vi "AO FIFO control.vi"(8 "NoOfSamples":u16, 9 "PulseEnd":u16, 10 "Counter":u16, 11 "PulseStart":u16) -> ()   [LabVIEW 2015]
uses:
  <vilib>/rvi/DataTransferAndStorage/Container/XNode/niFpgaContainer.xnode
  <vilib>/eio/EIONode/EIONode.xnode
  <vilib>/rvi/FIFO/Fifo_Resource/nirvififoEmulationWrite.vi
  <vilib>/rvi/eio/common/nirviEmuTemplateMethod_errors.vi
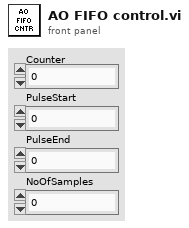
[diagram p1: front panel]
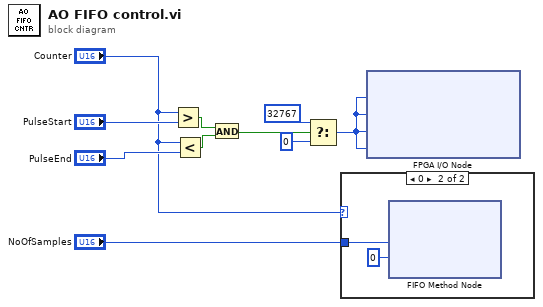
[diagram p0: block diagram]
diagram:
  n1 = Greater?(x="Counter", y="PulseStart") -> (0:w9:bool)
  n2 = Less?(x="Counter", y="PulseEnd") -> (x < y?=w10:bool)
  n3 = And(x=w9, y=w10) -> (x .and. y?=w6:bool)
  n4 = Select(t=i16 32767 ("IO Module\\AO 0 N"), s=w6, f=i16 0) -> (s? t:f=w4:i16)
  n5 = case shown="0" "Counter" {
    tunnel: "NoOfSamples" -> [_ w11]
    frame Default {
    }
    frame 0 {
      n6 = xnode ("FIFO Method Node")("Element"=w11, "Timeout"=0) -> ()  [unwired: 1 in, 2 out]
    }
  }
  n7 = xnode "FPGA I/O Node"("IO Module\\AO 0 N-3"=w4, "IO Module\\AO 0 N-2"=w4, "IO Module\\AO 0 N-1"=w4, "IO Module\\AO 0 N"=w4) -> ()  [unwired: 4 in, 4 out]
